vi "Joystick Get3-19-14 535pm.vi"(8 "reset":bool, 9 "JoystickRefDrive 2":T2, 10 "JoystickRefOp":T2, 11 "JoystickRefDrive":T2) -> ()   [LabVIEW 2013]
uses:
  <vilib>/Rock Robotics/WPI/Joystick/WPI_JoystickDevRef.ctl
  <vilib>/Rock Robotics/WPI/Joystick/WPI_JoystickDeviceEnum.ctl
  AxisLayoutOpJoyReg.ctl
  ButtonLayoutOpJoyReg.ctl
  ButtonLayoutDriveJoyReg.ctl
  Events.vi
  <vilib>/addons/control/pid/pid.llb/PID (DBL).vi
  <vilib>/ptbypt/NI_PtbyPt.lvlib
  <vilib>/addons/control/pid/NI_PID_pid.lvlib
panel:
  in  "Increase value":dbl=4.2 format="%#_13g"
  in  "PID gains":T1={"proportional gain (Kc)"=1.0, "integral time (Ti, min)"=0.01, "derivative time (Td, min)"=0.0} {"derivative time (Td, min)" format="%.3f"; "integral time (Ti, min)" format="%.3f"; "proportional gain (Kc)" format="%.3f"}
  in  "Correct\nangle":bool
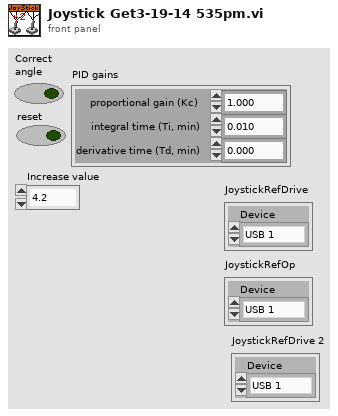
[diagram p1: front panel]
types:
  T1 = cluster{"proportional gain (Kc)":dbl, "integral time (Ti, min)":dbl, "derivative time (Td, min)":dbl}
  T2 = typedef "WPI_JoystickDevRef.ctl" = cluster{"Device":T3}
  T3 = typedef "WPI_JoystickDeviceEnum.ctl" = enum16{"USB 1", "USB 2", "USB 3", "USB 4", "Kinect 1", "Kinect 2"}
  T4 = typedef "ButtonLayoutDriveJoyReg.ctl" = cluster{"Ring light":bool, "Button 2":bool, "Button 3":bool, "Button 4":bool, "ShiftLow":bool, "ShiftHigh":bool, "Button 7":bool, "Button 8":bool, " Recalibrate":bool, "Exponential drive":bool, "Button 11":bool, "Button 12":bool}
  T5 = typedef "ButtonLayoutOpJoyReg.ctl" = cluster{"Accq Shoulder":bool, "Reload":bool, "Manuall truss servo":bool, "Button 4":bool, "Pass":bool, "Grab":bool, "Trajectory ctl":bool, "Throw":bool, "Accq Shoulder up":bool, "Button 10":bool, "Button 11":bool, "Button 12":bool}
  T6 = typedef "AxisLayoutOpJoyReg.ctl" = cluster{"axis 1":dbl, "axis 2":dbl, "axis 3":dbl, "axis 4":dbl, "axis 5":dbl, "Change Power":dbl}
  T7 = cluster{"OpJoyType":string, "DriveJoyType":string}
  T8 = cluster{"Translate":dbl, "Y-Axis (Backward Speed)":dbl, "Rotate":dbl, "Tank right side":dbl, "axis 5":dbl, "axis 6":dbl, "Use gyro":bool, "Exponential\ndrive":bool, "Ring light":bool}
  T9 = typedef "WPI_JoystickButtonState.ctl" = cluster{"Button 1":bool, "Button 2":bool, "Button 3":bool, "Button 4":bool, "Button 5":bool, "Button 6":bool, "Button 7":bool, "Button 8":bool, "Button 9":bool, "Button 10":bool, "Button 11":bool, "Button 12":bool}
  T10 = cluster{"axis 1 (x)":dbl, "axis 2 (y)":dbl, "axis 3 (throttle)":dbl, "axis 4":dbl, "axis 5":dbl, "axis 6":dbl}
  T11 = typedef "WPI_SolenoidValue.ctl" = enum16{"Off", "On", "Forward", "Reverse"}
  T12 = cluster{"Ultrasonic Distance (In)":dbl, "Gyro":dbl, "TopAquisition sensor":bool, "Encoder distance":dbl, "Encoder rate":dbl, "Encoder direction":bool, "winch engaged?":T11, "Motor Values":dbl[], "Latch encoder":u32, "BottomAquistion":bool, "BottomAquistion 2":bool, "Gyro Rate":dbl}
  T13 = cluster{"axis 1":dbl, "axis 2":dbl, "axis 3":dbl, "axis 4":dbl, "axis 5":dbl, "Change Power":dbl}
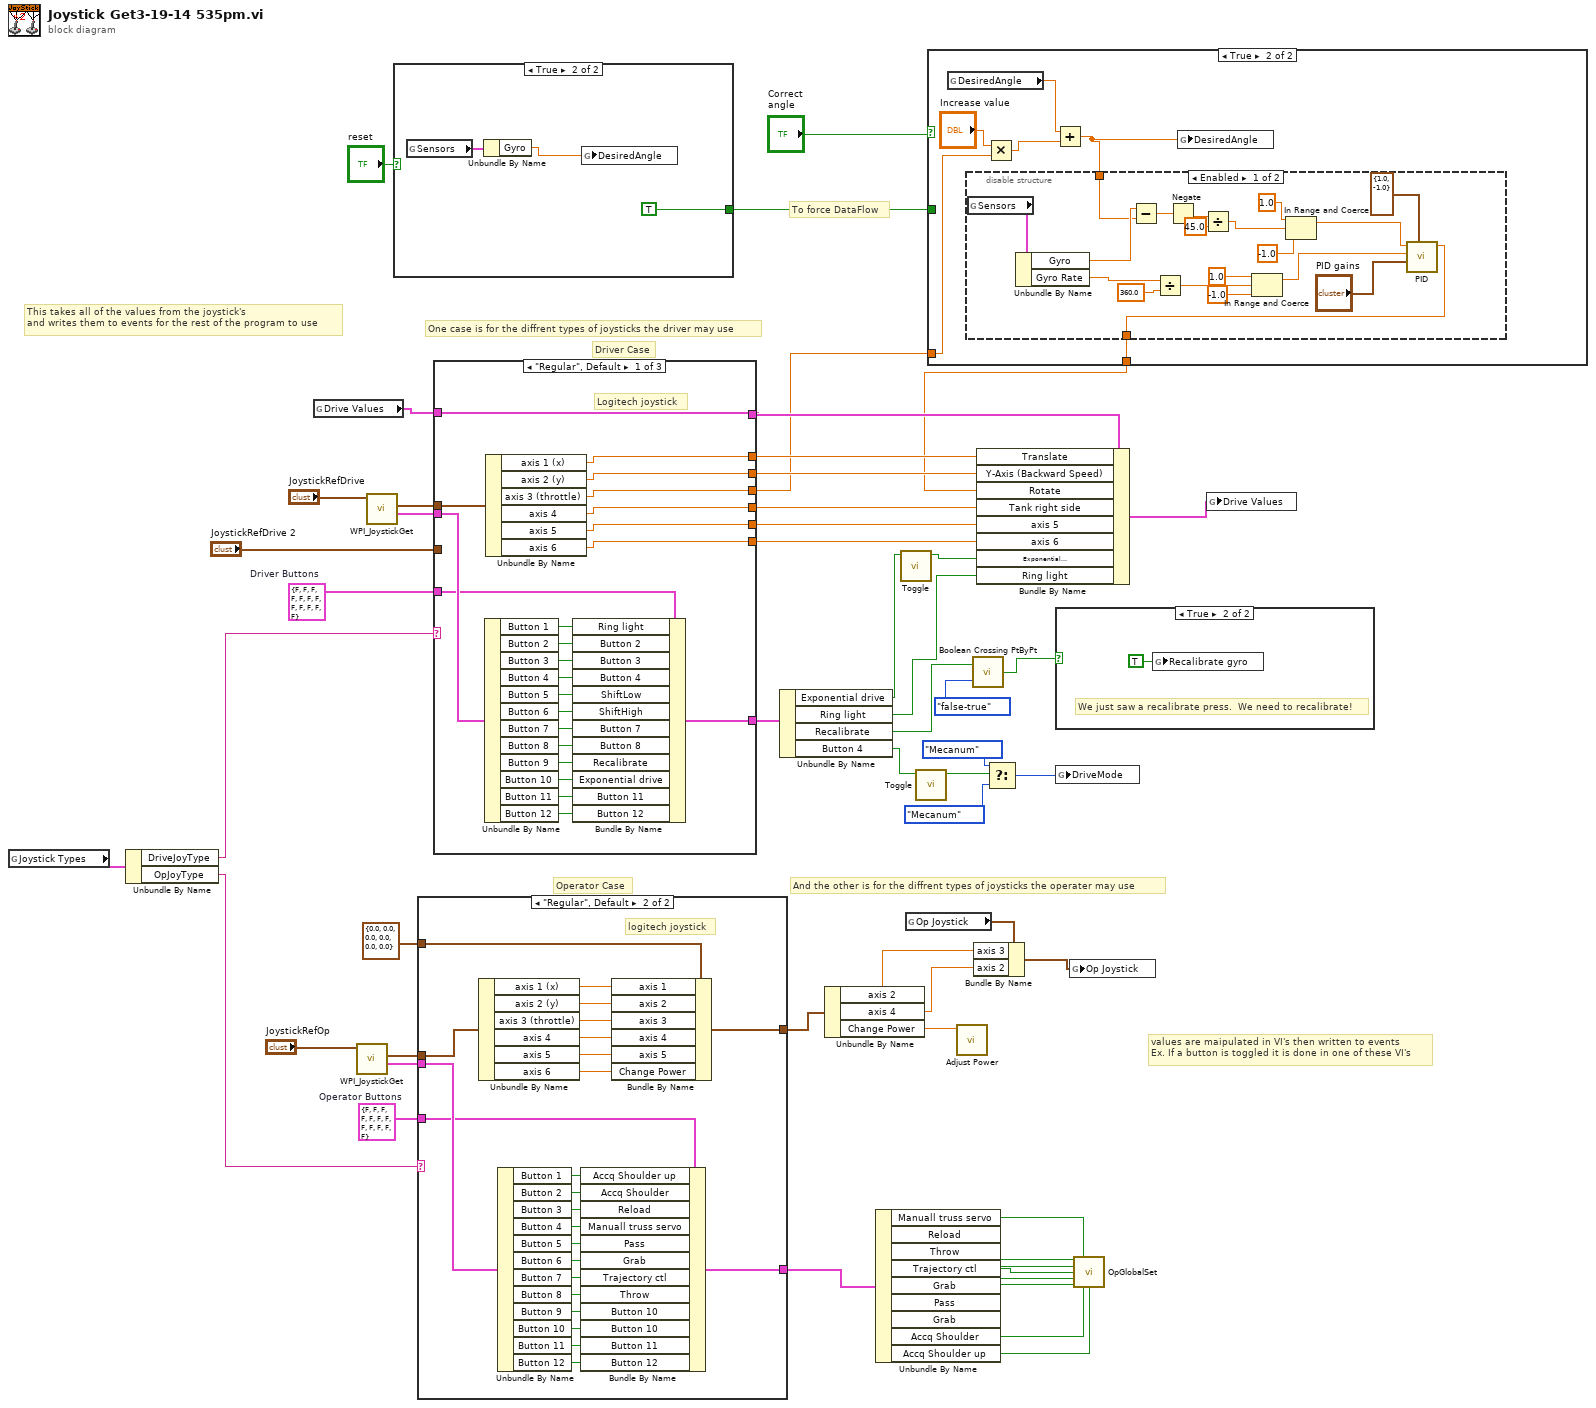
[diagram p0: block diagram]
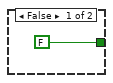
[diagram p2: hidden frame]
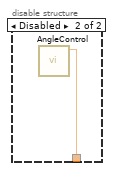
[diagram p4: hidden frame]
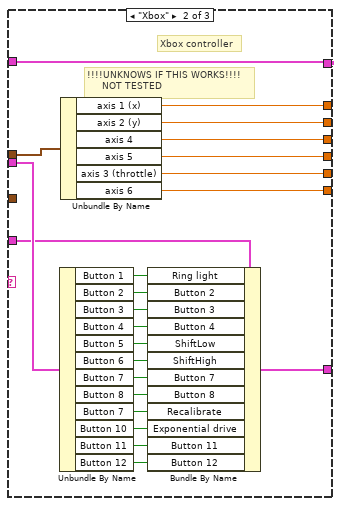
[diagram p6: hidden frame]
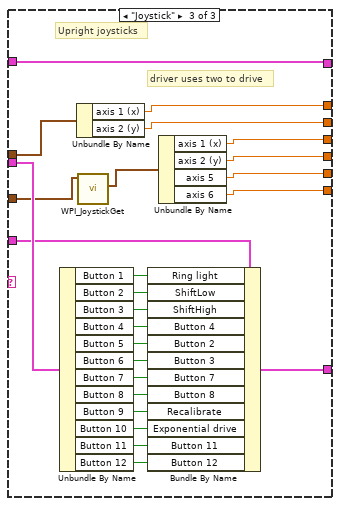
[diagram p7: hidden frame]
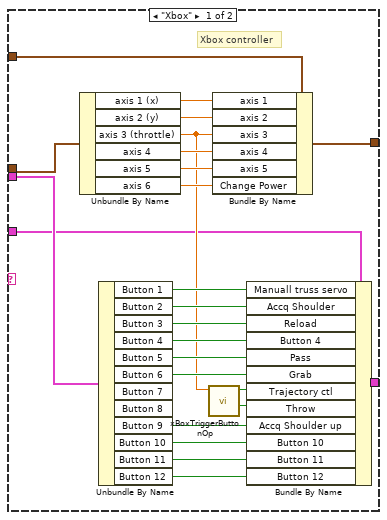
[diagram p8: hidden frame]
diagram:
  w36 = T4 {"Ring light"=FALSE, "Button 2"=FALSE, "Button 3"=FALSE, "Button 4"=FALSE, "ShiftLow"=FALSE, "ShiftHigh"=FALSE, "Button 7"=FALSE, "Button 8"=FALSE, " Recalibrate"=FALSE, "Exponential drive"=FALSE, "Button 11"=FALSE, "Button 12"=FALSE}  # Driver Buttons
  w37 = T5 {"Accq Shoulder"=FALSE, "Reload"=FALSE, "Manuall truss servo"=FALSE, "Button 4"=FALSE, "Pass"=FALSE, "Grab"=FALSE, "Trajectory ctl"=FALSE, "Throw"=FALSE, "Accq Shoulder up"=FALSE, "Button 10"=FALSE, "Button 11"=FALSE, "Button 12"=FALSE}  # Operator Buttons
  # "To force DataFlow"
  # "values are maipulated in VI's then written to events\nEx. If a button is toggled it is done in one of these VI's"
  # "And the other is for the diffrent types of joysticks the operater may use"
  # "One case is for the diffrent types of joysticks the driver may use"
  # "This takes all of the values from the joystick's\nand writes them to events for the rest of the program to use"
  # "Operator Case"
  # "Driver Case"
  n1 = global read "Events.vi" "Joystick Types"() -> (w35:T7)
  n2 = Unbundle By Name(w35) -> ("DriveJoyType"=w12:string, "OpJoyType"=w11:string)
  n3 = global read "Events.vi" "Drive Values"() -> (w34:T8)
  n4 = call <vilib>:"WPI_JoystickGet.vi"("JoystickDevRef"="JoystickRefOp") -> ("Buttons"=w48:T9, "Axes"=w47:T10)  [unwired: 4 in, 1 out]
  n5 = call <vilib>:"WPI_JoystickGet.vi"("JoystickDevRef"="JoystickRefDrive") -> ("Buttons"=w52:T9, "Axes"=w51:T10)  [unwired: 4 in, 1 out]
  n6 = case shown="True" "reset" {
    tunnel: [FALSE TRUE] -> w1
    frame False {
    }
    frame True {
      n7 = global read "Events.vi" "Sensors"() -> (w57:T12)
      n8 = Unbundle By Name(w57) -> ("Gyro"=w55:dbl)
      n9 = global write "Events.vi" "DesiredAngle"(w55) -> ()
    }
  }
  n10 = case shown="\"Regular\", Default" w11 {
    tunnel: w48 -> [w65 w93]
    tunnel: w47 -> [w66 w92]
    tunnel: [w64 w85] -> w46
    tunnel: [w63 w84] -> w39
    tunnel: T6 {"axis 1"=0.0, "axis 2"=0.0, "axis 3"=0.0, "axis 4"=0.0, "axis 5"=0.0, "Change Power"=0.0} ("input cluster") -> [w58 w83]
    tunnel: w37 -> [w59 w82]
    frame "Xbox" {
      # "Xbox controller"
      n11 = Unbundle By Name(w66) -> ("axis 1 (x)"=w71:dbl, "axis 2 (y)"=w70:dbl, "axis 3 (throttle)"=w60:dbl, "axis 4"=w69:dbl, "axis 5"=w68:dbl, "axis 6"=w67:dbl)
      n12 = Unbundle By Name(w65) -> ("Button 1"=w81:bool, "Button 2"=w80:bool, "Button 3"=w79:bool, "Button 4"=w78:bool, "Button 5"=w77:bool, "Button 6"=w76:bool, "Button 9"=w75:bool, "Button 10"=w74:bool, "Button 11"=w73:bool, "Button 12"=w72:bool)  [unwired: 2 out]
      n13 = call "xBoxTriggerButtonOp.vi"("zAxis"=w60) -> ("Throw"=w61:bool, "Lob"=w62:bool)  [unwired: 9 in]
      n14 = Bundle By Name(cluster=w58, "axis 1"=w71, "axis 2"=w70, "axis 3"=w60, "axis 4"=w69, "axis 5"=w68, "Change Power"=w67) -> (w64:T6)
      n15 = Bundle By Name(cluster=w59, "Manuall truss servo"=w81, "Accq Shoulder"=w80, "Reload"=w79, "Button 4"=w78, "Pass"=w77, "Grab"=w76, "Trajectory ctl"=w62, "Throw"=w61, "Accq Shoulder up"=w75, "Button 10"=w74, "Button 11"=w73, "Button 12"=w72) -> (w63:T5)
    }
    frame "Regular", Default {
      # "logitech joystick"
      n16 = Unbundle By Name(w92) -> ("axis 1 (x)"=w91:dbl, "axis 2 (y)"=w90:dbl, "axis 3 (throttle)"=w89:dbl, "axis 4"=w88:dbl, "axis 5"=w87:dbl, "axis 6"=w86:dbl)
      n17 = Unbundle By Name(w93) -> ("Button 1"=w105:bool, "Button 2"=w104:bool, "Button 3"=w103:bool, "Button 4"=w102:bool, "Button 5"=w101:bool, "Button 6"=w100:bool, "Button 7"=w99:bool, "Button 8"=w98:bool, "Button 9"=w97:bool, "Button 10"=w96:bool, "Button 11"=w95:bool, "Button 12"=w94:bool)
      n18 = Bundle By Name(cluster=w82, "Accq Shoulder up"=w105, "Accq Shoulder"=w104, "Reload"=w103, "Manuall truss servo"=w102, "Pass"=w101, "Grab"=w100, "Trajectory ctl"=w99, "Throw"=w98, "Button 10"=w97, "Button 10"=w96, "Button 11"=w95, "Button 12"=w94) -> (w84:T5)
      n19 = Bundle By Name(cluster=w83, "axis 1"=w91, "axis 2"=w90, "axis 3"=w89, "axis 4"=w88, "axis 5"=w87, "Change Power"=w86) -> (w85:T6)
    }
  }
  n20 = case shown="\"Regular\", Default" w12 {
    tunnel: w52 -> [w128 w151 w176]
    tunnel: w51 -> [w127 w150 w175]
    tunnel: [w112 w132 w160] -> w33
    tunnel: [w114 w137 w162] -> w50
    tunnel: w34 -> [w112 w132 w160]
    tunnel: w36 -> [w113 w136 w161]
    tunnel: [w111 w135 w159] -> w19
    tunnel: [w110 w134 w158] -> w32
    tunnel: [w109 w129 w157] -> w5
    tunnel: [w108 w130 w156] -> w31
    tunnel: [w107 w131 w155] -> w30
    tunnel: [w106 w133 w154] -> w29
    tunnel: "JoystickRefDrive 2" -> [_ _ w153]
    frame "Regular", Default {
      # "Logitech joystick"
      n21 = Unbundle By Name(w128) -> ("Button 1"=w126:bool, "Button 2"=w125:bool, "Button 3"=w124:bool, "Button 4"=w123:bool, "Button 5"=w122:bool, "Button 6"=w121:bool, "Button 7"=w120:bool, "Button 8"=w119:bool, "Button 9"=w118:bool, "Button 10"=w117:bool, "Button 11"=w116:bool, "Button 12"=w115:bool)
      n22 = Unbundle By Name(w127) -> ("axis 1 (x)"=w111:dbl, "axis 2 (y)"=w110:dbl, "axis 3 (throttle)"=w109:dbl, "axis 4"=w108:dbl, "axis 5"=w107:dbl, "axis 6"=w106:dbl)
      n23 = Bundle By Name(cluster=w113, "Ring light"=w126, "Button 2"=w125, "Button 3"=w124, "Button 4"=w123, "ShiftLow"=w122, "ShiftHigh"=w121, "Button 7"=w120, "Button 8"=w119, "Recalibrate"=w118, "Exponential drive"=w117, "Button 11"=w116, "Button 12"=w115) -> (w114:T4)
    }
    frame "Xbox" {
      # "Xbox controller"
      # "!!!!UNKNOWS IF THIS WORKS!!!!\n     NOT TESTED"
      n24 = Unbundle By Name(w151) -> ("Button 1"=w149:bool, "Button 2"=w148:bool, "Button 3"=w147:bool, "Button 4"=w146:bool, "Button 5"=w145:bool, "Button 6"=w144:bool, "Button 7"=w143:bool, "Button 8"=w142:bool, "Button 7"=w141:bool, "Button 10"=w140:bool, "Button 11"=w139:bool, "Button 12"=w138:bool)
      n25 = Unbundle By Name(w150) -> ("axis 1 (x)"=w135:dbl, "axis 2 (y)"=w134:dbl, "axis 4"=w129:dbl, "axis 5"=w130:dbl, "axis 3 (throttle)"=w131:dbl, "axis 6"=w133:dbl)
      n26 = Bundle By Name(cluster=w136, "Ring light"=w149, "Button 2"=w148, "Button 3"=w147, "Button 4"=w146, "ShiftLow"=w145, "ShiftHigh"=w144, "Button 7"=w143, "Button 8"=w142, "Recalibrate"=w141, "Exponential drive"=w140, "Button 11"=w139, "Button 12"=w138) -> (w137:T4)
    }
    frame "Joystick" {
      # "driver uses two to drive"
      # "Upright joysticks"
      n27 = Unbundle By Name(w176) -> ("Button 1"=w174:bool, "Button 2"=w173:bool, "Button 3"=w172:bool, "Button 4"=w171:bool, "Button 5"=w170:bool, "Button 6"=w169:bool, "Button 7"=w168:bool, "Button 8"=w167:bool, "Button 9"=w166:bool, "Button 10"=w165:bool, "Button 11"=w164:bool, "Button 12"=w163:bool)
      n28 = Unbundle By Name(w175) -> ("axis 1 (x)"=w159:dbl, "axis 2 (y)"=w158:dbl)
      n29 = call <vilib>:"WPI_JoystickGet.vi"("JoystickDevRef"=w153) -> ("Axes"=w152:T10)  [unwired: 4 in, 2 out]
      n30 = Bundle By Name(cluster=w161, "Ring light"=w174, "ShiftLow"=w173, "ShiftHigh"=w172, "Button 4"=w171, "Button 2"=w170, "Button 3"=w169, "Button 7"=w168, "Button 8"=w167, "Recalibrate"=w166, "Exponential drive"=w165, "Button 11"=w164, "Button 12"=w163) -> (w162:T4)
      n31 = Unbundle By Name(w152) -> ("axis 1 (x)"=w157:dbl, "axis 2 (y)"=w156:dbl, "axis 5"=w155:dbl, "axis 6"=w154:dbl)
    }
  }
  n32 = Unbundle By Name(w50) -> ("Exponential drive"=w17:bool, "Ring light"=w14:bool, "Recalibrate"=w28:bool, "Button 4"=w10:bool)
  n33 = Unbundle By Name(w46) -> ("axis 2"=w13:dbl, "axis 4"=w20:dbl, "Change Power"=w45:dbl)
  n34 = Unbundle By Name(w39) -> ("Manuall truss servo"=w16:bool, "Reload"=w44:bool, "Throw"=w43:bool, "Trajectory ctl"=w42:bool, "Grab"=w41:bool, "Pass"=w40:bool, "Accq Shoulder"=w23:bool, "Accq Shoulder up"=w15:bool)  [unwired: 1 out]
  n35 = call "Toggle.vi"("input"=w17) -> ("output"=w18:bool)  [unwired: 10 in]
  n36 = global read "Events.vi" "Op Joystick"() -> (w22:T13)
  n37 = call "Toggle.vi"("input"=w10) -> ("output"=w9:bool)  [unwired: 10 in]
  n38 = case shown="True" "Correct\nangle" {
    tunnel: w5 -> [w177 w179]
    tunnel: [w177 w178] -> w4
    tunnel: w1 -> [_ _]
    frame False {
    }
    frame True {
      n39 = global read "Events.vi" "DesiredAngle"() -> (w183:dbl)
      n40 = Multiply(x="Increase value", y=w179) -> (x*y=w182:dbl)
      n41 = Add(x=w183, y=w182) -> (x+y=w180:dbl)
      n42 = disable-structure shown="Enabled" {
        disable-tunnel: w180 -> [w200 _]
        disable-tunnel: [w185 w203] -> w178
        frame Enabled {
          n43 = global read "Events.vi" "Sensors"() -> (w202:T12)
          n44 = Unbundle By Name(w202) -> ("Gyro"=w201:dbl, "Gyro Rate"=w193:dbl)
          n45 = Subtract(x=w201, y=w200) -> (x-y=w199:dbl)
          n46 = Divide(x=w193, y=360.0) -> (x/y=w189:dbl)
          n47 = Negate(x=w199) -> (-x=w198:dbl)
          n48 = Divide(x=w198, y=45.0) -> (x/y=w194:dbl)
          n49 = In Range and Coerce(upper limit=1.0, x=w189, lower limit=-1.0) -> (coerced(x)=w187:dbl)  [unwired: 1 out]
          n50 = In Range and Coerce(upper limit=1.0, x=w194, lower limit=-1.0) -> (coerced(x)=w186:dbl)  [unwired: 1 out]
          n51 = call-poly <vilib>:"PID.vi"("output range"=cluster{"output high":dbl, "output low":dbl} {"output high"=1.0, "output low"=-1.0}, "PID gains"="PID gains", "process variable"=w187, "setpoint"=w186) -> ("output"=w185:dbl)  [unwired: 6 in, 1 out]
        }
        frame Disabled {
          n52 = call "AngleControl.vi"() -> ("motor"=w203:dbl)  [unwired: 11 in]
        }
      }
      n53 = global write "Events.vi" "DesiredAngle"(w180) -> ()
    }
  }
  n54 = call "Adjust Power.vi"("D-pad input"=w45) -> ()  [unwired: 11 in]
  n55 = call <vilib>:"Boolean Crossing PtByPt.vi"("direction"=enum16{"either", "false-true", "true-false"}."false-true", "input"=w28) -> ("crossing"=w25:bool)  [unwired: 1 in]
  n56 = Bundle By Name(cluster=w22, "axis 3"=w13, "axis 2"=w20) -> (w21:T13)
  n57 = Bundle By Name(cluster=w33, "Translate"=w19, "Y-Axis (Backward Speed)"=w32, "Rotate"=w4, "Tank right side"=w31, "axis 5"=w30, "axis 6"=w29, "Exponential\ndrive"=w18, "Ring light"=w14) -> (w24:T8)
  n58 = Select(t=enum16{"Arcade", "Tank", "Mecanum"}."Mecanum" ("DriveMode"), s=w9, f=enum16{"Arcade", "Tank", "Mecanum"}."Mecanum" ("DriveMode")) -> (s? t:f=w8:enum16{"Arcade", "Tank", "Mecanum"})
  n59 = case shown="True" w25 {
    frame False {
      # "We don't know that we don't need to recalibrate.\nDon't change anything."
    }
    frame True {
      # "We just saw a recalibrate press.  We need to recalibrate!"
      n60 = global write "Events.vi" "Recalibrate gyro"(TRUE ("Recalibrate gyro")) -> ()
    }
  }
  n61 = global write "Events.vi" "DriveMode"(w8) -> ()
  n62 = global write "Events.vi" "Op Joystick"(w21) -> ()
  n63 = call "OpGlobalSet.vi"("ReloadButton"=w44, "Manuall servo"=w16, "ThrowButton"=w43, "LobButton"=w42, "GrabButton"=w41, "GroundPassButton"=w40, "Shoulder joint"=w23, "Shoulder joint up"=w15) -> ()  [unwired: 8 in]
  n64 = global write "Events.vi" "Drive Values"(w24) -> ()
